vi "Get settings chain.vi"(8 "error in (no error)":errorcluster, 11 "StageSPIMBase in":refnum<class "StageSPIM.lvclass">) -> (0 "error out":errorcluster, 1 "class name":string[](array[string]), 2 "settings":variant[](array[variant]), 3 "StageSPIMBase out":refnum<class "StageSPIM.lvclass">)   [LabVIEW 2012, in "StageSPIM.lvclass"]
doc: "Returns an array of variants containing the settings clusters of each class in the inheritance chain (lowest child class first), together with an array of all class names in the inheritance chain.\n\nFor classes without settings cluster, the settings chain contains empty variants."
uses:
  StageSPIM.lvclass
  <vilib>/Distrio/Murmex/Murmex/Murmex.lvclass
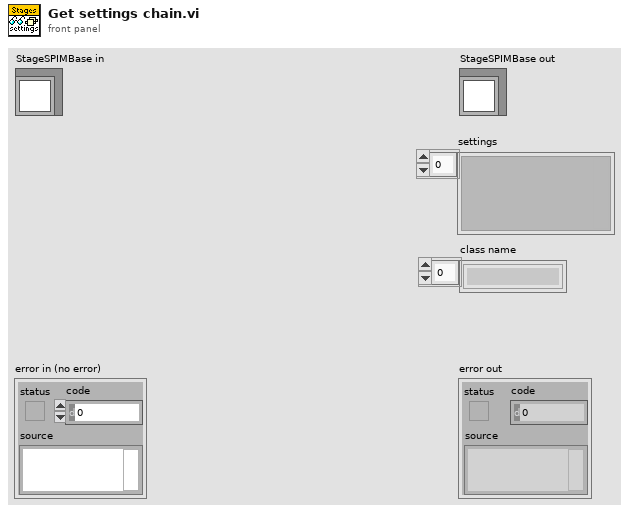
[diagram p1: front panel]
types:
  T1 = typedef "StageSPIM.lvclass/settings_cluster.ctl" = cluster{"speedA":dbl[unit], "speedX":dbl[unit], "speedY":dbl[unit], "speedZ":dbl[unit], "speedFocus":dbl[unit]}
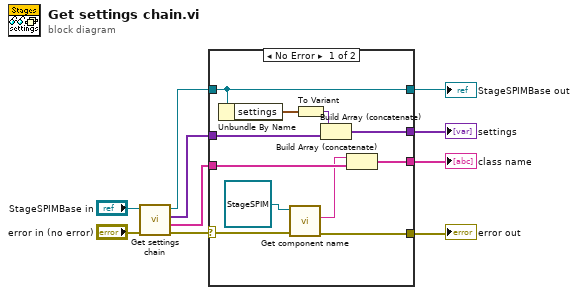
[diagram p0: block diagram]
diagram:
  n1 = call-parent "Get settings chain.vi"("error in (no error)"="error in (no error)", "MurmexBase in"="StageSPIMBase in") -> ("error out"=w8:errorcluster, "class name"=w2:string[], "settings"=w4:variant[], "MurmexBase out"=w6:refnum<class "StageSPIM.lvclass">)  [unwired: 6 in]
  n2 = case shown="No Error" w8 {
    selector: w8 -> [w21 w22]
    tunnel: [w20 w22] -> w7
    tunnel: w6 -> [w11 w25]
    tunnel: [w11 w25] -> w5
    tunnel: w4 -> [w16 w24]
    tunnel: [w15 w24] -> w3
    tunnel: w2 -> [w14 w23]
    tunnel: [w12 w23] -> w1
    frame No Error {
      n3 = Unbundle By Name(w11) -> ("settings"=w17:T1)
      n4 = call <vilib>:"Get component name.vi"("error in (no error)"=w21, "Murmex in"=refnum<class "StageSPIM.lvclass"> refnum ("StageSPIM.lvclass")) -> ("error out"=w20:errorcluster, "component name"=w13:string)  [unwired: 7 in, 1 out]
      n5 = To Variant(anything=w17) -> (Variant=w18:variant)
      n6 = Build Array (concatenate)(w18, w16) -> (w15:variant[])
      n7 = Build Array (concatenate)(w13, w14) -> (w12:string[])
    }
    frame Error {
    }
  }
  "error out" <- w7
  "StageSPIMBase out" <- w5
  "settings" <- w3
  "class name" <- w1
